vi "Test Coffee Shop Customer Submit Order Sent to Waiting to Order Queue.vi"(8 "error in (no error)":errorcluster, 11 "Coffee Shop Test in":refnum<class "Coffee Shop Test.lvclass">) -> (0 "error out":errorcluster, 3 "Coffee Shop Test out":refnum<class "Coffee Shop Test.lvclass">)   [LabVIEW 2020, in "Coffee Shop Test.lvclass"]
uses:
  Coffee Shop Test.lvclass
  C:/Program Files (x86)/National Instruments/LabVIEW 2020/vi.lib/Astemes/LUnit/Test Case.lvclass
  Processes/Coffee Shop/Coffee Shop.lvclass
  C:/Program Files (x86)/National Instruments/LabVIEW 2020/vi.lib/Astemes/Triarc Framework/Process/Process.lvclass
  C:/Program Files (x86)/National Instruments/LabVIEW 2020/vi.lib/Astemes/Triarc Framework/Application/Application.lvclass
  Test Doubles/Mock Job Handler/Mock Job Handler.lvclass
  C:/git/astemes-triarc-examples/source/Coffee Shop/Processes/People/Process Job/Job Handler.lvclass
  Processes/People/Customers/Customer/Customer.lvclass
  Support/Beverages/TypeDefs/Drink Type.ctl
  Support/Beverages/TypeDefs/Options.ctl
  <vilib>/Astemes/Triarc Framework/Process/Process.lvclass/Process.ctl
  <vilib>/Astemes/Triarc Framework/Application/Application.lvclass/Application.ctl
  <vilib>/Astemes/Triarc Framework/Synchronous Request Callback/Synchronous Request Callback.lvclass/Synchronous Request Callback.ctl
  <vilib>/Astemes/LUnit/Test Case.lvclass/Test Case.ctl
  <vilib>/Astemes/Triarc Framework/Process/Public/Lifecycle/Get Lifecycle State.vi
  <vilib>/Astemes/Triarc Framework/Application/Private/Retrieve Process from App.vi
  <vilib>/Astemes/Triarc Framework/Application/Private/Parse Process Name.vi
  <vilib>/Astemes/Triarc Framework/Application/Private/Get Process from Map.vi
  <vilib>/Astemes/Triarc Framework/Process/Private/SubVIs/Wait for finish.vi
  <vilib>/Astemes/Triarc Framework/Process/Private/SubVIs/Set Lifecycle State.vi
  <vilib>/Astemes/Triarc Framework/Process/Protected/Messaging/Send Message.vi
  <vilib>/Astemes/LUnit/Append Pass Result.vi
  <vilib>/Astemes/LUnit/Append Fail Result.vi
  <vilib>/Utility/error.llb/Clear Errors.vi
  <vilib>/Astemes/Triarc Framework/Process/Protected/Messaging/Request Message.vi
  <vilib>/Astemes/Triarc Framework/Application/Private/Add Process to Map.vi
  <vilib>/AdvancedString/Delimited String to 1D String Array.vi
  <vilib>/Astemes/Triarc Framework/Process/Private/SubVIs/Handle Debug Data.vi
  <vilib>/Astemes/Triarc Framework/Synchronous Request Callback/Create.vi
  <vilib>/Astemes/Triarc Framework/Process/Protected/Messaging/Async Request Message.vi
  <vilib>/Astemes/Triarc Framework/Logging/Log Debug.vi
  <vilib>/AdvancedString/1D String Array to Delimited String.vi
  <vilib>/Utility/High Resolution Relative Seconds.vi
  <vilib>/Astemes/Triarc Framework/Application/Application.lvclass
  <vilib>/Astemes/Triarc Framework/Synchronous Request Callback/Synchronous Request Callback.lvclass
  C:/Program Files (x86)/National Instruments/LabVIEW 2020/vi.lib/Astemes/Triarc Framework/Callback/Callback.lvclass
  <vilib>/Astemes/Triarc Framework/Process/Process.lvclass
  C:/Program Files (x86)/National Instruments/LabVIEW 2020/vi.lib/Astemes/Triarc Framework/Logging/Logging.lvclass
  <vilib>/Astemes/Triarc Framework/Process/Public/Read Name.vi
  <vilib>/Utility/error.llb/Error Cluster From Error Code.vi
  <vilib>/Astemes/Triarc Framework/Process/Private/SubVIs/Wait for Response Message.vi
  <vilib>/Astemes/Triarc Framework/Callback/Callback.lvclass
  <vilib>/Astemes/Triarc Framework/Logging/Logging.lvclass
  Support/Beverages/Beverage/Beverage.lvclass
  <vilib>/Astemes/LUnit/Test Case.lvclass
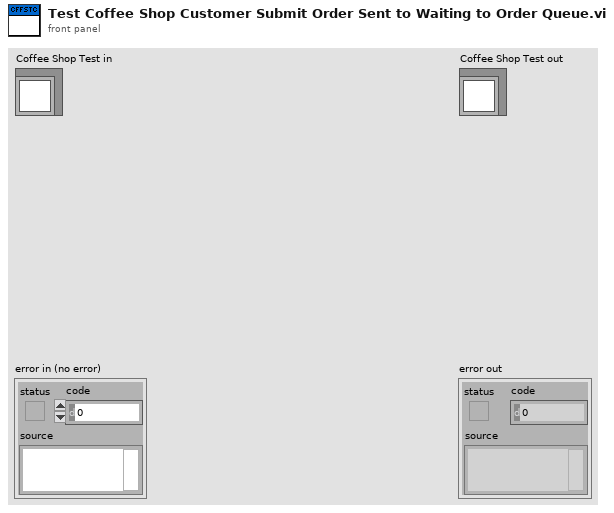
[diagram p1: front panel]
types:
  T1 = typedef "Beverage.lvclass/Drink Type.ctl" = enum16{"Dark Roast", "Decaf", "Espresso", "House Blend"}
  T2 = typedef "Beverage.lvclass/Options.ctl" = enum16{"<None>", "Milk", "Mocha", "Soy", "Whip"}
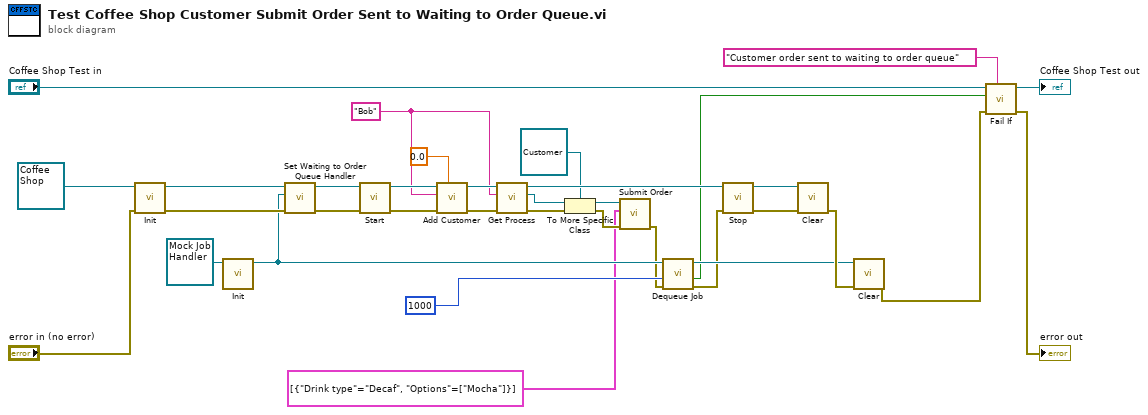
[diagram p0: block diagram]
diagram:
  w9 = "Bob" ("Name")
  n1 = call-dynamic "Init.vi"("error in (no error)"="error in (no error)", "Process In"=refnum<class "Coffee Shop.lvclass"> refnum ("Coffee Shop.lvclass")) -> ("error out"=w34:errorcluster, "Process Out"=w27:refnum<class "Coffee Shop.lvclass">)  [unwired: 8 in]
  n2 = call-dynamic "Init.vi"("Mock Job Handler In"=refnum<class "Mock Job Handler.lvclass"> refnum) -> ("Mock Job Handler Out"=w21:refnum<class "Mock Job Handler.lvclass">)  [unwired: 9 in, 1 out]
  n3 = call "Set Waiting to Order Queue Handler.vi"("error in (no error)"=w34, "Waiting To Order Queue Handler"=w21, "Coffee Shop In"=w27) -> ("error out"=w32:errorcluster, "Coffee Shop Out"=w33:refnum<class "Coffee Shop.lvclass">)  [unwired: 7 in]
  n4 = call <vilib>:"Start.vi"("error in (no error)"=w32, "Process In"=w33) -> ("error out"=w31:errorcluster, "Process Out"=w26:refnum<class "Coffee Shop.lvclass">)  [unwired: 7 in, 1 out]
  n5 = call "Add Customer.vi"("Time scale [ms]"=0.0 ("Delay Before Leaving [s]"), "error in (no error)"=w31, "Name"=w9, "Coffee Shop in"=w26) -> ("error out"=w24:errorcluster, "Coffee Shop out"=w11:refnum<class "Coffee Shop.lvclass">)  [unwired: 6 in]
  n6 = call <vilib>:"Get Process.vi"("error in (no error)"=w24, "Process Name"=w9, "Application In"=w11) -> ("error out"=w12:errorcluster, "App Process"=w8:refnum<class "Process.lvclass">, "Application Out"=w10:refnum<class "Coffee Shop.lvclass">)  [unwired: 6 in]
  n7 = To More Specific Class(target class=refnum<class "Customer.lvclass"> refnum ("Customer.lvclass"), reference=w8, error in=w12) -> (specific class reference=w6:refnum<class "Customer.lvclass">, error out=w5:errorcluster)
  n8 = call "Submit Order.vi"("error in (no error)"=w5, "Order Content"=cluster{"Drink type":T1, "Options":T2[]}[] [{"Drink type"=enum."Decaf", "Options"=[enum."Mocha"]}], "Customer In"=w6) -> ("error out"=w4:errorcluster)  [unwired: 7 in, 1 out]
  n9 = call "Dequeue Job.vi"("error in (no error)"=w4, "timeout in ms (-1)"=1000, "Mock Job Handler In"=w21) -> ("error out"=w14:errorcluster, "timed out?"=w2:bool, "Mock Job Handler Out"=w22:refnum<class "Mock Job Handler.lvclass">)  [unwired: 5 in, 1 out]
  n10 = call <vilib>:"Stop.vi"("error in (no error)"=w14, "Process In"=w10) -> ("error out"=w29:errorcluster, "Process Out"=w30:refnum<class "Coffee Shop.lvclass">)  [unwired: 7 in, 1 out]
  n11 = call-dynamic "Clear.vi"("error in (no error)"=w29, "Application In"=w30) -> ("error out"=w23:errorcluster)  [unwired: 9 in]
  n12 = call-dynamic "Clear.vi"("error in (no error)"=w23, "Mock Job Handler In"=w22) -> ("error out"=w16:errorcluster)  [unwired: 9 in]
  n13 = call <vilib>:"Fail If.vi"("Description"="Customer order sent to waiting to order queue", "error in (no error)"=w16, "Fail?"=w2, "LUnit Test Case In"="Coffee Shop Test in") -> ("error out"=→"error out":errorcluster, "LUnit Test Case Out"=→"Coffee Shop Test out":refnum<class "Coffee Shop Test.lvclass">)  [unwired: 6 in]
